vi "Write Key (Raw).vi"(7 "Section Name":string, 8 "error in (no error)":errorcluster, 9 "Content":string, 10 "Key Name":string, 11 "Config in":refnum<class "LabVIEW-Config.lvclass">) -> (0 "error out":errorcluster, 2 "Key Replaced?":bool, 3 "Config out":refnum<class "LabVIEW-Config.lvclass">)   [LabVIEW 2017, in "LabVIEW-Config.lvlib" / "LabVIEW-Config.lvclass"]
uses:
  LabVIEW-Config.lvclass
  LabVIEW-Config.lvclass/LabVIEW-Config.ctl
  LineToken.ctl
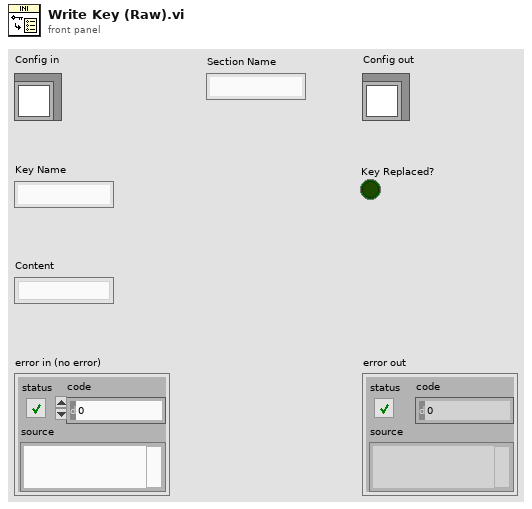
[diagram p1: front panel]
types:
  T1 = typedef "LabVIEW-Config.lvlib/LabVIEW-Config.lvclass/LineToken.ctl" = enum8{"comment", "section", "key", "more"}
  T2 = typedef "LabVIEW-Config.lvlib/LabVIEW-Config.lvclass/KeyInfo.ctl" = cluster{"Key Indexes":cluster{"Indexes":i32[]}[], "Session Found?":bool, "Key found?":bool, "Session Index":i32}
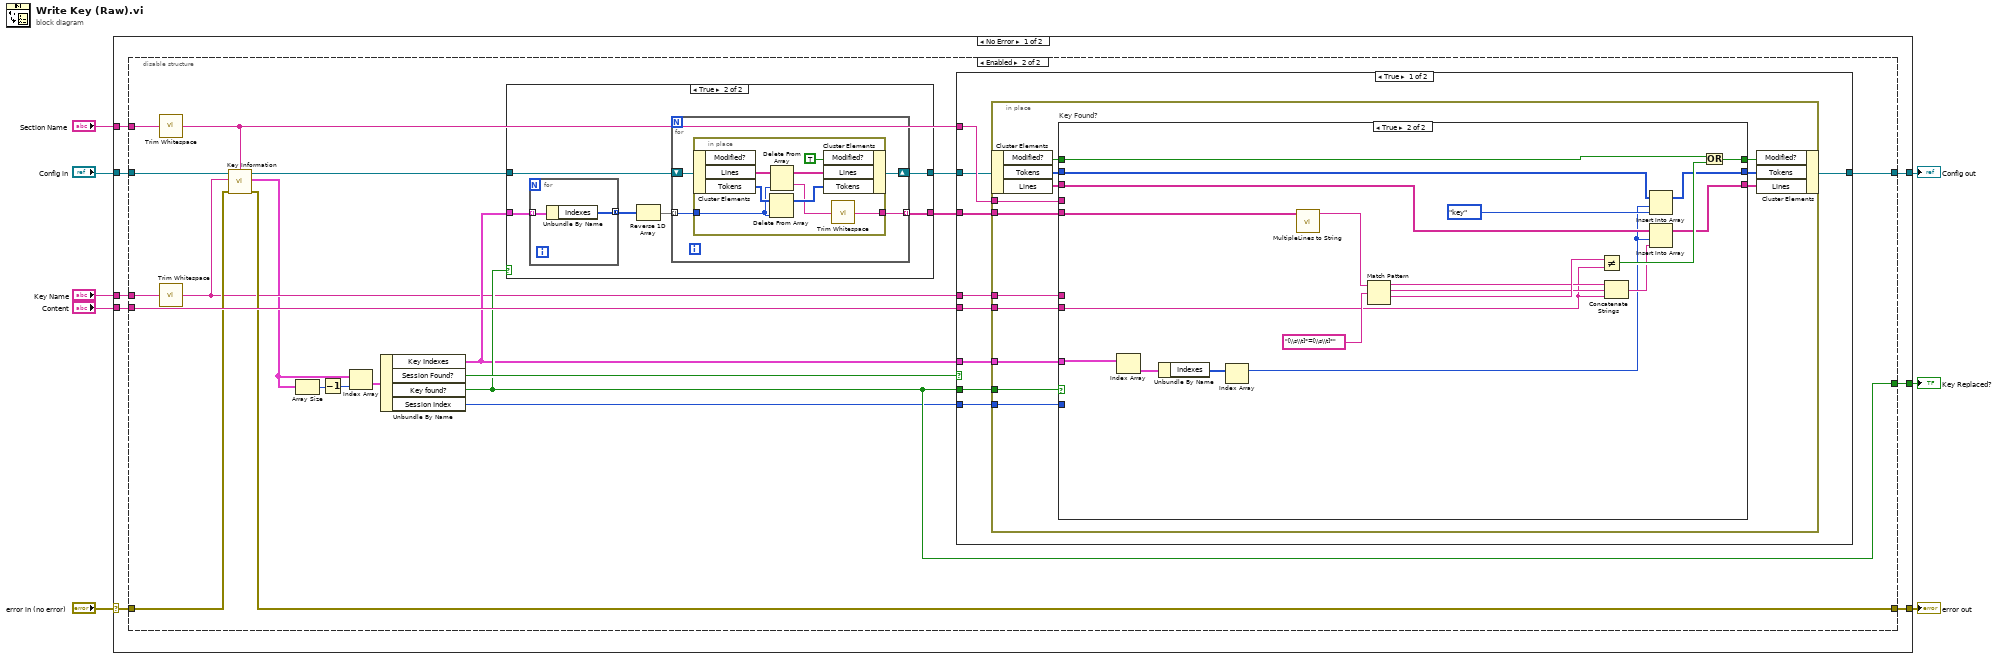
[diagram p0: block diagram]
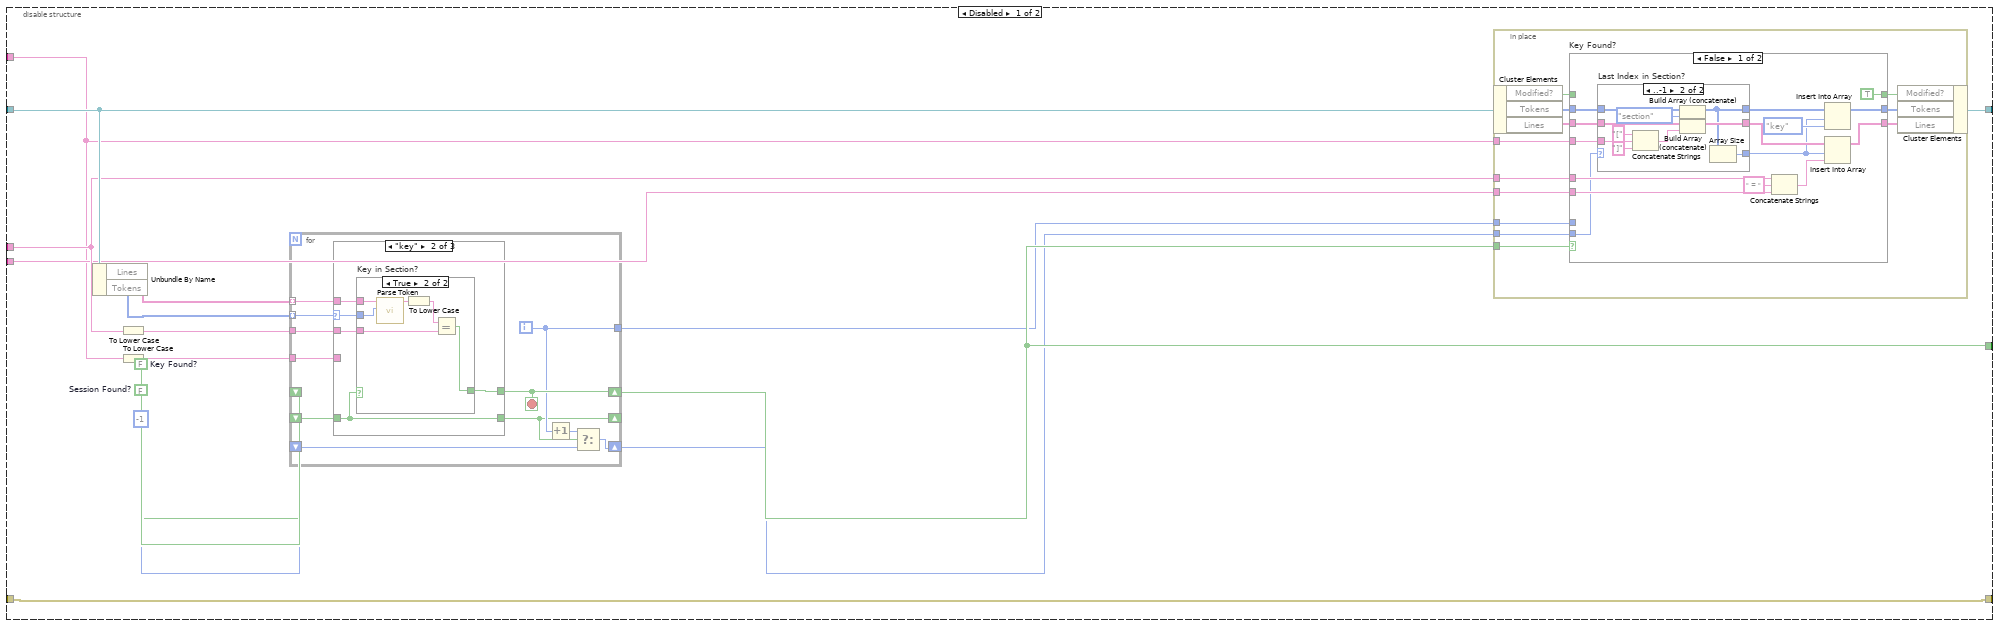
[diagram p2: hidden frame]
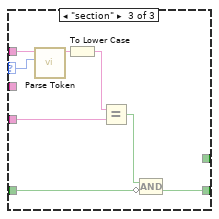
[diagram p5: hidden frame]
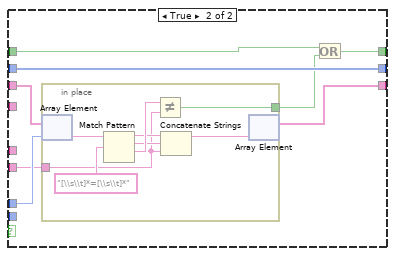
[diagram p7: hidden frame]
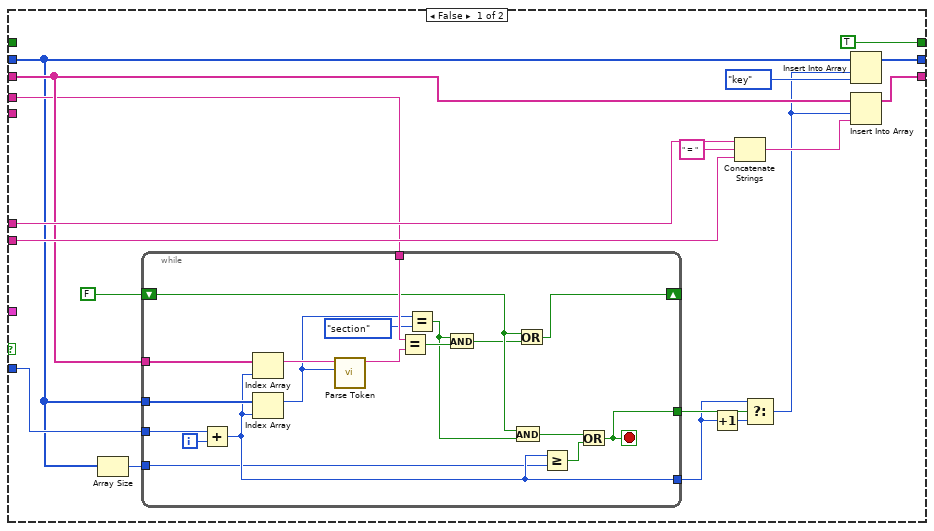
[diagram p9: hidden frame]
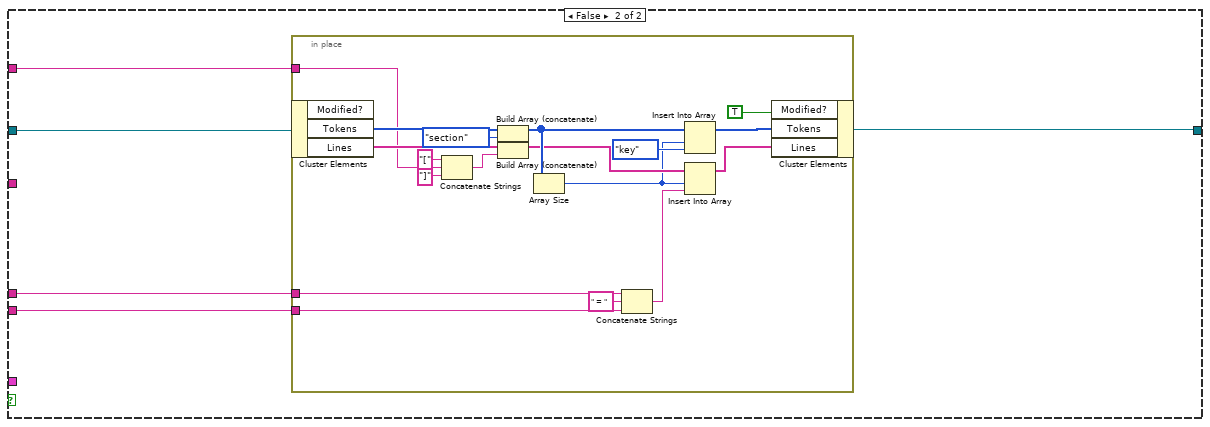
[diagram p10: hidden frame]
diagram:
  n1 = case shown="No Error" "error in (no error)" {
    selector: "error in (no error)" -> [w10 w264]
    tunnel: "Config in" -> [w15 w263]
    tunnel: [w9 w264] -> w7
    tunnel: [w11 w263] -> w5
    tunnel: "Section Name" -> [w12 _]
    tunnel: [w16 _] -> w3
    tunnel: "Key Name" -> [w14 _]
    tunnel: "Content" -> [w13 _]
    frame No Error {
      n2 = disable-structure shown="Enabled" {
        disable-tunnel: [w26 w129] -> w16
        disable-tunnel: w15 -> [w24 w137]
        disable-tunnel: w14 -> [w21 w135]
        disable-tunnel: w13 -> [w20 w139]
        disable-tunnel: w12 -> [w19 w136]
        disable-tunnel: [w18 w138] -> w11
        disable-tunnel: w10 -> [w17 w134]
        disable-tunnel: [w17 w133] -> w9
        frame Disabled {
          w28 = FALSE  # Key Found?
          w29 = FALSE  # Session Found?
          n3 = Unbundle By Name(w24) -> ("Lines"=w31:string[], "Tokens"=w32:T1[])
          n4 = To Lower Case(string=w21) -> (all lower case string=w27:string)
          n5 = To Lower Case(string=w19) -> (all lower case string=w30:string)
          n6 = for {
            tunnel: w32 -> [w43] mode=indexing
            tunnel: w31 -> [w42] mode=indexing
            tunnel: w30 -> [w41]
            shift-right: [w33] -> _
            shift-left: w29 -> [w35]
            shift-right: [w39] -> w26
            shift-left: w28 -> [_]
            tunnel: w27 -> [w40]
            tunnel: [w38] -> w23
            shift-right: [w37] -> w22
            shift-left: -1 -> [w36]
            i -> [w38]
            stop <- w39 stop-if-true
            n7 = case shown="\"key\"" w43 {
              selector: w43 -> [_ w45 w56]
              tunnel: w42 -> [_ w49 w58]
              tunnel: w41 -> [_ _ w63]
              tunnel: [w44 w48 w59] -> w33
              tunnel: w35 -> [w44 w48 w61]
              tunnel: w40 -> [_ w47 _]
              tunnel: [_ w46 _] -> w39
              frame "comment" {
              }
              frame "key" {
                n8 = case "Key in Section?" shown="True" w48 {
                  tunnel: w49 -> [_ w52]
                  tunnel: w47 -> [_ w55]
                  tunnel: [_ w53] -> w46
                  tunnel: w45 -> [_ w51]
                  frame False {
                  }
                  frame True {
                    n9 = call "Parse Token.vi"("Token"=w51, "Line"=w52) -> ("Name"=w50:string)  [unwired: 8 in, 1 out]
                    n10 = To Lower Case(string=w50) -> (all lower case string=w54:string)
                    n11 = Equal?(x=w54, y=w55) -> (x = y?=w53:bool)
                  }
                }
              }
              frame "section" {
                n12 = call "Parse Token.vi"("Token"=w56, "Line"=w58) -> ("Name"=w57:string)  [unwired: 8 in, 1 out]
                n13 = To Lower Case(string=w57) -> (all lower case string=w62:string)
                n14 = Equal?(x=w62, y=w63) -> (x = y?=w60:bool)
                n15 = Compound Arithmetic op=AND(w60, invert w61) -> (w59:bool)
              }
            }
            n16 = Increment(x=w38) -> (x+1=w34:i32)
            n17 = Select(t=w34, s=w33, f=w36) -> (s? t:f=w37:i32)
          }
          n18 = in-place {
            in-place-border: w26 -> [w75]
            in-place-border: w23 -> [w68]
            in-place-border: w22 -> [w67]
            in-place-border: w21 -> [w66]
            in-place-border: w20 -> [w65]
            in-place-border: w19 -> [w64]
            n19 = in-place-cluster #1(w24) -> ("Modified?"=w70:bool, "Tokens"=w74:T1[], "Lines"=w73:string[])
            n20 = case "Key Found?" shown="False" w75 {
              tunnel: w74 -> [w89 w110]
              tunnel: w73 -> [w88 w109]
              tunnel: [w86 w110] -> w72
              tunnel: [w87 w108] -> w71
              tunnel: w70 -> [_ w104]
              tunnel: [TRUE ("Modified?") w105] -> w69
              tunnel: w67 -> [w76 _]
              tunnel: w66 -> [w85 _]
              tunnel: w65 -> [w84 w107]
              tunnel: w64 -> [w78 _]
              tunnel: w68 -> [_ w111]
              frame False {
                n21 = case "Last Index in Section?" shown="..-1" w76 {
                  selector: w76 -> [w91 _]
                  tunnel: w89 -> [w93 w96]
                  tunnel: w88 -> [w92 w103]
                  tunnel: [w93 w94] -> w80
                  tunnel: [w92 w102] -> w79
                  tunnel: w78 -> [_ w100]
                  tunnel: [w91 w95] -> w77
                  frame 0.. {
                  }
                  frame ..-1 {
                    n22 = Concatenate Strings("[" ("string"), w100, "]" ("string")) -> (w97:string)
                    n23 = Build Array (concatenate)(w96, LineToken."section" ("new element/subarray")) -> (w94:T1[])
                    n24 = Build Array (concatenate)(w103, w97) -> (w102:string[])
                    n25 = Array Size(array=w94) -> (size(s)=w95:i32)
                  }
                }
                n26 = Concatenate Strings(w85, " = " ("string"), w84) -> (w81:string)
                n27 = Insert Into Array(array=w80, index=w77, new element=LineToken."key" ("new element/subarray")) -> (w86:T1[])
                n28 = Insert Into Array(array=w79, index=w77, new element=w81) -> (w87:string[])
              }
              frame True {
                n29 = in-place {
                  in-place-border: w107 -> [w114]
                  in-place-border: [w112] -> w106
                  n30 = in-place-array #2(w109, w111) -> (w118:string)
                  n31 = Match Pattern(string=w118, regular expression="[\\s\\t]*=[\\s\\t]*") -> (before substring=w116:string, match substring=w115:string, after substring=w117:string)  [unwired: 1 in, 1 out]
                  n32 = Not Equal?(x=w117, y=w114) -> (x != y?=w112:bool)
                  n33 = Concatenate Strings(w116, w115, w114) -> (w113:string)
                  n34 = in-place-array #2(w113) -> (w108:string[])  [unwired: 1 out]
                }
                n35 = Or(x=w104, y=w106) -> (x .or. y?=w105:bool)
              }
            }
            n36 = in-place-cluster #1("Modified?"=w69, "Tokens"=w72, "Lines"=w71) -> (w18:refnum<class "LabVIEW-Config.lvclass">)
          }
        }
        frame Enabled {
          n37 = call <vilib>:"Trim Whitespace.vi"("string"=w136) -> ("trimmed string"=w126:string)  [unwired: 1 in]
          n38 = call <vilib>:"Trim Whitespace.vi"("string"=w135) -> ("trimmed string"=w125:string)  [unwired: 1 in]
          n39 = call "Key Information.vi"("Section Name"=w126, "error in (no error)"=w134, "Key Name"=w125, "Config in"=w137) -> ("error out"=w133:errorcluster, "Key Information"=w122:T2[], "Config out"=w132:refnum<class "LabVIEW-Config.lvclass">)  [unwired: 5 in]
          n40 = Array Size(array=w122) -> (size(s)=w123:i32)
          n41 = Decrement(x=w123) -> (x-1=w121:i32)
          n42 = Index Array(array=w122, index=w121) -> (element=w124:T2)
          n43 = Unbundle By Name(w124) -> ("Key Indexes"=w128:cluster{"Indexes":i32[]}[], "Session Found?"=w130:bool, "Key found?"=w129:bool, "Session Index"=w120:i32)
          n44 = case shown="True" w129 {
            tunnel: w128 -> [_ w142]
            tunnel: w132 -> [w140 w146]
            tunnel: [w140 w145] -> w131
            tunnel: [_ w144] -> w127
            frame False {
            }
            frame True {
              n45 = for {
                tunnel: w142 -> [w148] mode=indexing
                tunnel: [w147] -> w141 mode=concatenating
                n46 = Unbundle By Name(w148) -> ("Indexes"=w147:i32[])
              }
              n47 = Reverse 1D Array(array=w141) -> (reversed array=w143:i32[])
              n48 = for {
                tunnel: w143 -> [w150] mode=indexing
                shift-right: [w152] -> w145
                shift-left: w146 -> [w151]
                tunnel: [w149] -> w144 mode=indexing
                n49 = in-place {
                  in-place-border: w150 -> [w155]
                  in-place-border: [w153] -> w149
                  n50 = in-place-cluster #3(w151) -> ("Lines"=w159:string[], "Tokens"=w158:T1[])  [unwired: 1 out]
                  n51 = Delete From Array(array=w158, index=w155) -> (array with subset deleted=w157:T1[])  [unwired: 1 in, 1 out]
                  n52 = Delete From Array(array=w159, index=w155) -> (deleted portion=w154:string, array with subset deleted=w156:string[])  [unwired: 1 in]
                  n53 = in-place-cluster #3("Modified?"=TRUE, "Lines"=w156, "Tokens"=w157) -> (w152:refnum<class "LabVIEW-Config.lvclass">)
                  n54 = call <vilib>:"Trim Whitespace.vi"("string"=w154) -> ("trimmed string"=w153:string)  [unwired: 1 in]
                }
              }
            }
          }
          n55 = case shown="True" w130 {
            tunnel: w139 -> [w169 w244]
            tunnel: [w168 w243] -> w138
            tunnel: w126 -> [w167 w242]
            tunnel: w125 -> [w166 w241]
            tunnel: w131 -> [w165 w240]
            tunnel: w129 -> [w164 _]
            tunnel: w128 -> [w163 _]
            tunnel: w127 -> [w162 _]
            tunnel: w120 -> [w161 _]
            frame True {
              n56 = in-place {
                in-place-border: w164 -> [w182]
                in-place-border: w166 -> [w175]
                in-place-border: w169 -> [w174]
                in-place-border: w167 -> [w173]
                in-place-border: w163 -> [w172]
                in-place-border: w162 -> [w171]
                in-place-border: w161 -> [w170]
                n57 = in-place-cluster #4(w165) -> ("Modified?"=w177:bool, "Tokens"=w181:T1[], "Lines"=w180:string[])
                n58 = case "Key Found?" shown="True" w182 {
                  tunnel: w181 -> [w184 w227]
                  tunnel: w180 -> [w192 w236]
                  tunnel: [w198 w226] -> w179
                  tunnel: [w199 w235] -> w178
                  tunnel: w177 -> [_ w237]
                  tunnel: [TRUE ("Modified?") w238] -> w176
                  tunnel: w175 -> [w197 _]
                  tunnel: w174 -> [w196 w229]
                  tunnel: w173 -> [w191 _]
                  tunnel: w172 -> [_ w230]
                  tunnel: w171 -> [_ w223]
                  tunnel: w170 -> [w185 _]
                  frame False {
                    n59 = Array Size(array=w184) -> (size(s)=w183:i32)
                    n60 = while {
                      tunnel: w192 -> [w219]
                      tunnel: w184 -> [w215]
                      tunnel: w191 -> [w216]
                      shift-right: [w213] -> _
                      shift-left: FALSE -> [w211]
                      tunnel: [w204] -> w188
                      tunnel: [w201] -> w189
                      tunnel: w185 -> [w206]
                      tunnel: w183 -> [w203]
                      i -> [w207]
                      stop <- w201 stop-if-true
                      n61 = Add(x=w206, y=w207) -> (x+y=w204:i32)
                      n62 = Index Array(array=w219, index=w204) -> (element=w209:string)
                      n63 = Index Array(array=w215, index=w204) -> (element=w208:T1)
                      n64 = call "Parse Token.vi"("Token"=w208, "Line"=w209) -> ("Name"=w218:string)  [unwired: 8 in, 1 out]
                      n65 = Equal?(x=w216, y=w218) -> (x = y?=w217:bool)
                      n66 = Equal?(x=w208, y=LineToken."section") -> (x = y?=w212:bool)
                      n67 = And(x=w212, y=w217) -> (x .and. y?=w210:bool)
                      n68 = And(x=w211, y=w212) -> (x .and. y?=w202:bool)
                      n69 = Or(x=w211, y=w210) -> (x .or. y?=w213:bool)
                      n70 = Greater Or Equal?(x=w204, y=w203) -> (x >= y?=w205:bool)
                      n71 = Or(x=w202, y=w205) -> (x .or. y?=w201:bool)
                    }
                    n72 = Increment(x=w188) -> (x+1=w186:i32)
                    n73 = Concatenate Strings(w197, " = " ("string"), w196) -> (w193:string)
                    n74 = Select(t=w188, s=w189, f=w186) -> (s? t:f=w187:i32)
                    n75 = Insert Into Array(array=w184, index=w187, new element=LineToken."key" ("new element/subarray")) -> (w198:T1[])
                    n76 = Insert Into Array(array=w192, index=w187, new element=w193) -> (w199:string[])
                  }
                  frame True {
                    n77 = Index Array(array=w230) -> (element=w225:cluster{"Indexes":i32[]})  [unwired: 1 in]
                    n78 = Unbundle By Name(w225) -> ("Indexes"=w221:i32[])
                    n79 = Index Array(array=w221) -> (element=w220:i32)  [unwired: 1 in]
                    n80 = call "MultipleLines to String.vi"("Array"=w223) -> ("String"=w222:string)  [unwired: 10 in]
                    n81 = Match Pattern(string=w222, regular expression="[\\s\\t]*=[\\s\\t]*") -> (before substring=w232:string, match substring=w231:string, after substring=w233:string)  [unwired: 1 in, 1 out]
                    n82 = Not Equal?(x=w233, y=w229) -> (x != y?=w239:bool)
                    n83 = Concatenate Strings(w232, w231, w229) -> (w228:string)
                    n84 = Insert Into Array(array=w227, index=w220, new element=LineToken."key" ("new element/subarray")) -> (w226:T1[])
                    n85 = Insert Into Array(array=w236, index=w220, new element=w228) -> (w235:string[])
                    n86 = Or(x=w237, y=w239) -> (x .or. y?=w238:bool)
                  }
                }
                n87 = in-place-cluster #4("Modified?"=w176, "Tokens"=w179, "Lines"=w178) -> (w168:refnum<class "LabVIEW-Config.lvclass">)
              }
            }
            frame False {
              n88 = in-place {
                in-place-border: w241 -> [w257]
                in-place-border: w244 -> [w256]
                in-place-border: w242 -> [w255]
                n89 = in-place-cluster #5(w240) -> ("Tokens"=w262:T1[], "Lines"=w261:string[])  [unwired: 1 out]
                n90 = Concatenate Strings("[" ("string"), w255, "]" ("string")) -> (w245:string)
                n91 = Build Array (concatenate)(w262, LineToken."section" ("new element/subarray")) -> (w251:T1[])
                n92 = Build Array (concatenate)(w261, w245) -> (w250:string[])
                n93 = Array Size(array=w251) -> (size(s)=w249:i32)
                n94 = Concatenate Strings(w257, " = " ("string"), w256) -> (w252:string)
                n95 = Insert Into Array(array=w251, index=w249, new element=LineToken."key" ("new element/subarray")) -> (w260:T1[])
                n96 = Insert Into Array(array=w250, index=w249, new element=w252) -> (w259:string[])
                n97 = in-place-cluster #5("Modified?"=TRUE, "Tokens"=w260, "Lines"=w259) -> (w243:refnum<class "LabVIEW-Config.lvclass">)
              }
            }
          }
        }
      }
    }
    frame Error {
    }
  }
  "error out" <- w7
  "Config out" <- w5
  "Key Replaced?" <- w3
